vi "Library_Sensors_init.vi"(8 "error in (no error)":errorcluster) -> (0 "error out":errorcluster)   [LabVIEW 2013]
uses:
  Sensors/IMU/IMU_Data_Type_Def.ctl
  My Computer/Controls/Sensors State.ctl
  My Computer/Controls/Estimated Position.ctl
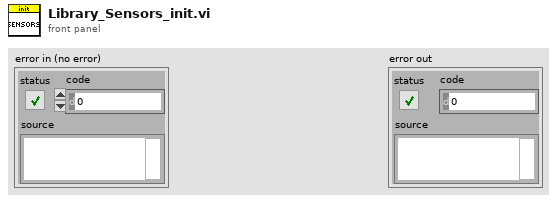
[diagram p1: front panel]
types:
  T1 = typedef "Estimated Position.ctl" = cluster{"X":dbl, "Y":dbl, "Z":dbl, "V_X":dbl, "V_Y":dbl, "V_Z":dbl}
  T2 = typedef "Sensors State.ctl" = cluster{"Leakage-Sensor_enabled":bool, "IMU_enabled":bool, "Swimbladder Fill-State-Sensor_enabled":bool, "Flow-Sensor_enabled":bool, "Depth-Sensor_enabled":bool, "Current-Sensor_enabled":bool, "Calibrate Depth":bool, "SB_Piston_Stuck_Detect_enabled":bool, "Check_too_Deep_enabled":bool}
  T3 = typedef "IMU_Data_Type_Def.ctl" = cluster{timestamp, "X_Gyro_Out":dbl, "Y_Gyro_Out":dbl, "Z_Gyro_Out":dbl, "X_Accl_Out":dbl, "Y_Accl_Out":dbl, "Z_Accl_Out":dbl, "X_Magn_Out":dbl, "Y_Magn_Out":dbl, "Z_Magn_Out":dbl, "Temp_Out":dbl, "Barom_Out":dbl}
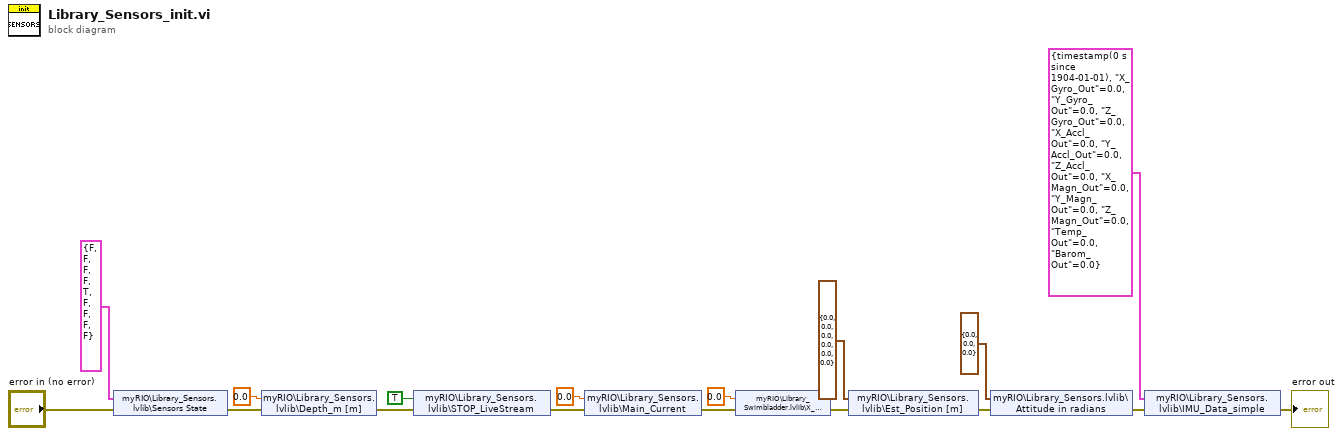
[diagram p0: block diagram]
diagram:
  n1 = shared-variable "myRIO\\Library_Sensors.lvlib\\Sensors State"(T2 {"Leakage-Sensor_enabled"=FALSE, "IMU_enabled"=FALSE, "Swimbladder Fill-State-Sensor_enabled"=FALSE, "Flow-Sensor_enabled"=FALSE, "Depth-Sensor_enabled"=TRUE, "Current-Sensor_enabled"=FALSE, "Calibrate Depth"=FALSE, "SB_Piston_Stuck_Detect_enabled"=FALSE, "Check_too_Deep_enabled"=FALSE} ("Sensors State"), error in="error in (no error)") -> (error out=w10:errorcluster)
  n2 = shared-variable "myRIO\\Library_Sensors.lvlib\\Depth_m [m]"(0.0 ("Depth [m]"), error in=w10) -> (error out=w9:errorcluster)
  n3 = shared-variable "myRIO\\Library_Sensors.lvlib\\STOP_LiveStream"(TRUE ("STOP_LiveStream"), error in=w9) -> (error out=w8:errorcluster)
  n4 = shared-variable "myRIO\\Library_Sensors.lvlib\\Main_Current"(0.0 ("Main_Current"), error in=w8) -> (error out=w7:errorcluster)
  n5 = shared-variable "myRIO\\Library_Swimbladder.lvlib\\X_desired"(0.0 ("coerced(x)"), error in=w7) -> (error out=w2:errorcluster)
  n6 = shared-variable "myRIO\\Library_Sensors.lvlib\\Est_Position [m]"(T1 {"X"=0.0, "Y"=0.0, "Z"=0.0, "V_X"=0.0, "V_Y"=0.0, "V_Z"=0.0} ("Est_Position [m]"), error in=w2) -> (error out=w1:errorcluster)
  n7 = shared-variable "myRIO\\Library_Sensors.lvlib\\Attitude in radians"(cluster{"Roll":dbl, "Pitch":dbl, "Yaw":dbl} {"Roll"=0.0, "Pitch"=0.0, "Yaw"=0.0} ("Attitude in degrees"), error in=w1) -> (error out=w6:errorcluster)
  n8 = shared-variable "myRIO\\Library_Sensors.lvlib\\IMU_Data_simple"(T3 {timestamp(0 s since 1904-01-01), "X_Gyro_Out"=0.0, "Y_Gyro_Out"=0.0, "Z_Gyro_Out"=0.0, "X_Accl_Out"=0.0, "Y_Accl_Out"=0.0, "Z_Accl_Out"=0.0, "X_Magn_Out"=0.0, "Y_Magn_Out"=0.0, "Z_Magn_Out"=0.0, "Temp_Out"=0.0, "Barom_Out"=0.0} ("IMU_Data_simple"), error in=w6) -> (error out=→"error out":errorcluster)
